vi "getArrayNotAssignedValueIdx.vi"(8 "error in (no error)":errorcluster, 9 "Assigned Value":dbl, 10 "Array":dbl[](array[numeric]), 11 "MatOper in":refnum<class "MatOper.lvclass">) -> (0 "error out":errorcluster, 2 "Index Array":i32[](array[numeric]), 3 "MatOper out":refnum<class "MatOper.lvclass">)   [LabVIEW 2016, in "OfcFunc.lvlib" / "MatOper.lvclass"]
doc: "Get the not-assigned-value index array. For example, if the input array is [0.0, 1.1, 2.2, 3.3] and the assigned value is 0, the output will be [1, 2, 3]."
uses:
  MatOper.lvclass
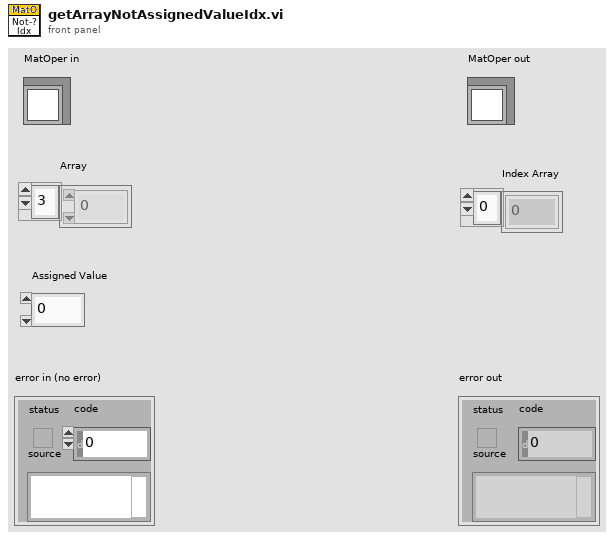
[diagram p1: front panel]
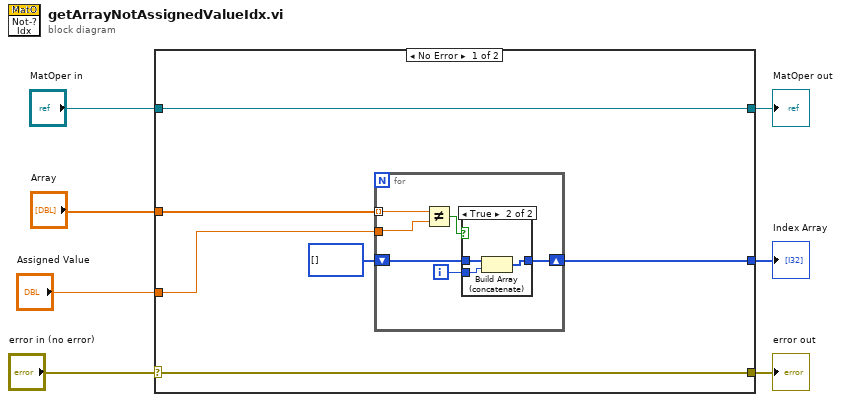
[diagram p0: block diagram]
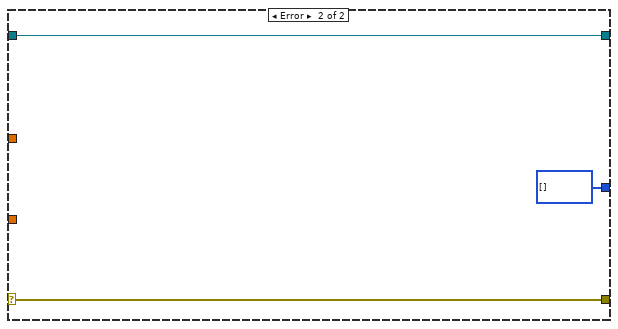
[diagram p3: hidden frame]
diagram:
  n1 = case shown="No Error" "error in (no error)" {
    selector: "error in (no error)" -> [w12 w26]
    tunnel: [w12 w26] -> w6
    tunnel: [w13 w25] -> w4
    tunnel: "MatOper in" -> [w13 w25]
    tunnel: "Array" -> [w10 _]
    tunnel: [w9 i32[] []] -> w2
    tunnel: "Assigned Value" -> [w8 _]
    frame No Error {
      n2 = for {
        tunnel: w10 -> [w18] mode=indexing
        shift-right: [w15] -> w9
        shift-left: i32[] [] -> [w16]
        tunnel: w8 -> [w14]
        i -> [w17]
        n3 = Not Equal?(x=w18, y=w14) -> (x != y?=w19:bool)
        n4 = case shown="True" w19 {
          tunnel: w17 -> [_ w23]
          tunnel: w16 -> [w20 w22]
          tunnel: [w20 w21] -> w15
          frame False {
          }
          frame True {
            n5 = Build Array (concatenate)(w22, w23) -> (w21:i32[])
          }
        }
      }
    }
    frame Error {
    }
  }
  "error out" <- w6
  "MatOper out" <- w4
  "Index Array" <- w2
